vi "XNET.Cluster.Initialize.vi"(8 "error in":errorcluster, 10 "CAN Cluster":T1={"Baud Rate"=125000, "Comment"="", "Name"=""}, 11 "database in":refnum<k21>) -> (0 "error out":errorcluster, 3 "cluster out":refnum<k21>)   [LabVIEW 2015, in "Diagnostics Addon Engine.lvlib"]
uses:
  Diagnostics Addon Engine.lvlib
  Types/XNET.Cluster.ctl
  <vilib>/xnet/xnet.llb/XNET Database Create (Cluster).vi
  <resource>/objmgr/xnet.rc
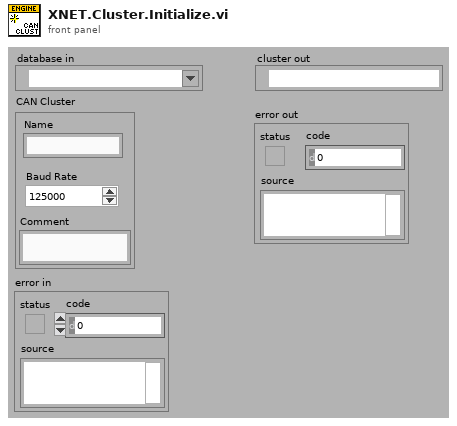
[diagram p1: front panel]
types:
  T1 = typedef "Diagnostics Addon Engine.lvlib/XNET.Cluster.ctl" = cluster{"Baud Rate":u32, "Comment":string, "Name":string}
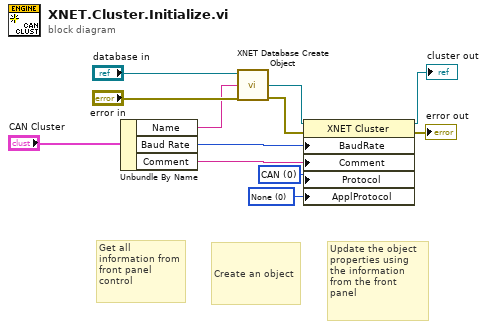
[diagram p0: block diagram]
diagram:
  w1 = u32 0 items=["None", "J1939"] ("Application Protocol")
  w12 = u32 0 items=["CAN", "FlexRay"] ("Protocol")
  # "Update the object properties using the information from the front panel"
  # "Create an object"
  # "Get all information from front panel control"
  n1 = Unbundle By Name("CAN Cluster") -> ("Name"=w7:string, "Baud Rate"=w8:u32, "Comment"=w9:string)
  n2 = call-poly <vilib>:"XNET Database Create Object.vi"("database in"="database in", "cluster name"=w7, "error in (no error)"="error in") -> ("cluster out"=w2:refnum<k21>, "error out"=w6:errorcluster)  [unwired: 10 in, 1 out]
  n3 = property class="XNET Cluster"(reference=w2, error in=w6, "BaudRate"=w8, "Comment"=w9, "Protocol"=w12, "ApplProtocol"=w1) -> (reference out=→"cluster out":refnum<k21>, error out=→"error out":errorcluster)
